vi "PolyCopyDocumentation.vi"   [LabVIEW 2020]
types:
  T1 = cluster{"VIPath":path, "Menu Name":string, "Selector Name":string}[]
  T2 = cluster{"vi reference":refnum<vi>, "Ctrls[]":refnum<vi>[]}
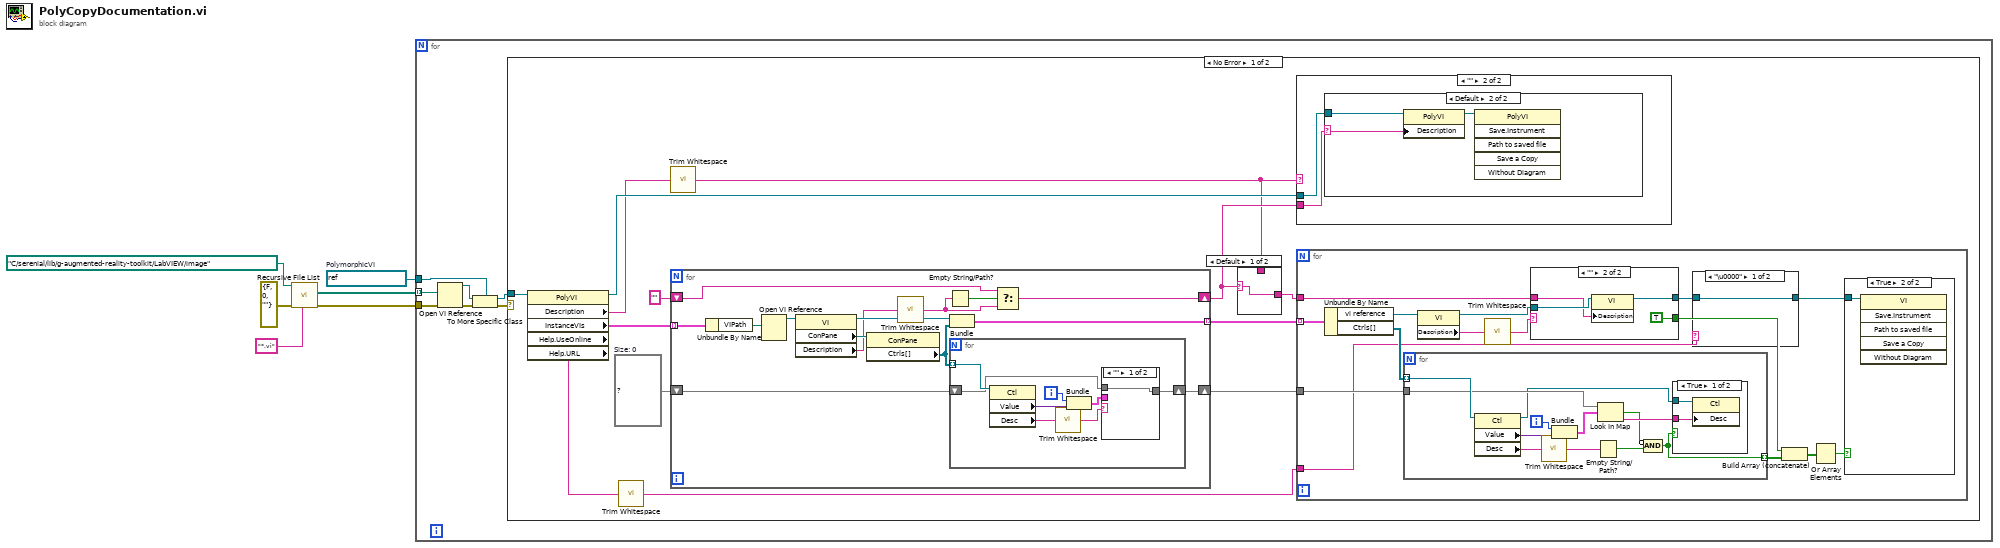
[diagram p0: block diagram]
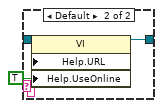
[diagram p5: hidden frame]
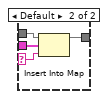
[diagram p9: hidden frame]
diagram:
  w3 = refnum<vi> refnum  # PolymorphicVI
  n1 = call <vilib>:"Recursive File List.vi"("pattern"="*.vi", "error in (no error)"=errorcluster {"status"=FALSE, "code"=0, "source"=""} ("error out"), "Folder Path"=path "C:/serenial/lib/g-augmented-reality-toolkit/LabVIEW/image") -> ("error out"=w6:errorcluster, "All Files in Dir"=w5:path[])  [unwired: 4 in, 3 out]
  n2 = for {
    tunnel: w6 -> [w13]
    tunnel: w5 -> [w12] mode=indexing
    tunnel: w3 -> [w11]
    n3 = Open VI Reference(vi path=w12, error in (no error)=w13) -> (vi reference=w10:refnum<vi>, error out=w9:errorcluster)  [unwired: 4 in]
    n4 = To More Specific Class(target class=w11, reference=w10, error in=w9) -> (specific class reference=w7:refnum<vi>, error out=w8:errorcluster)
    n5 = case shown="No Error" w8 {
      tunnel: w7 -> [w26 _]
      frame No Error {
        w25 = map{cluster{i32, "Value":variant}, string} {}  # Size: 0
        n6 = property class="PolyVI" props=["Description", "InstanceVIs", "Help.UseOnline", "Help.URL"](reference=w26) -> (reference out=w21:refnum<vi>, "Description"=w19:string, "InstanceVIs"=w20:T1, "Help.URL"=w15:string)  [unwired: 1 in, 2 out]
        n7 = call <vilib>:"Trim Whitespace.vi"("string"=w15) -> ("trimmed string"=w14:string)  [unwired: 1 in]
        n8 = call <vilib>:"Trim Whitespace.vi"("string"=w19) -> ("trimmed string"=w16:string)  [unwired: 1 in]
        n9 = for {
          tunnel: w20 -> [w87] mode=indexing
          shift-right: [w84] -> w22
          shift-left: w25 -> [w83]
          shift-right: [w75] -> w18
          shift-left: "" ("Description") -> [w77]
          tunnel: [w74] -> w23 mode=indexing
          n10 = Unbundle By Name(w87) -> ("VIPath"=w82:path)
          n11 = Open VI Reference(vi path=w82) -> (vi reference=w86:refnum<vi>)  [unwired: 5 in, 1 out]
          n12 = property class="VI"(reference=w86) -> (reference out=w81:refnum<vi>, "ConPane"=w85:refnum<vi>, "Description"=w79:string)  [unwired: 1 in, 1 out]
          n13 = property class="ConPane"(reference=w85) -> ("Ctrls[]"=w80:refnum<vi>[])  [unwired: 1 in, 2 out]
          n14 = call <vilib>:"Trim Whitespace.vi"("string"=w79) -> ("trimmed string"=w76:string)  [unwired: 1 in]
          n15 = Empty String/Path?(string/path=w76) -> (empty?=w78:bool)
          n16 = Bundle("vi reference"=w81, "Ctrls[]"=w80) -> (w74:T2)  [unwired: 1 in]
          n17 = for {
            tunnel: w80 -> [w95] mode=indexing
            shift-right: [w89] -> w84
            shift-left: w83 -> [w88]
            i -> [w93]
            n18 = property class="Ctl"(reference=w95) -> ("Value"=w94:variant, "Desc"=w91:string)  [unwired: 1 in, 2 out]
            n19 = call <vilib>:"Trim Whitespace.vi"("string"=w91) -> ("trimmed string"=w90:string)  [unwired: 1 in]
            n20 = Bundle(w93, "Value"=w94) -> (w92:cluster{i32, "Value":variant})  [unwired: 1 in]
            n21 = case shown="\"\"" w90 {
              selector: w90 -> [_ w99]
              tunnel: w92 -> [_ w100]
              tunnel: [w96 w98] -> w89
              tunnel: w88 -> [w96 w97]
              frame "" {
              }
              frame Default {
                n22 = Insert Into Map(map in=w97, key=w100, value=w99) -> (map out=w98:map{cluster{i32, "Value":variant}, string})  [unwired: 2 out]
              }
            }
          }
          n23 = Select(t=w77, s=w78, f=w76) -> (s? t:f=w75:string)
        }
        n24 = case shown="Default" w18 {
          selector: w18 -> [w27 _]
          tunnel: [w27 w28] -> w17
          tunnel: w16 -> [_ w28]
          frame Default {
          }
          frame "" {
          }
        }
        n25 = case shown="\"\"" w16 {
          tunnel: w21 -> [_ w30]
          tunnel: w18 -> [_ w29]
          frame Default {
          }
          frame "" {
            n26 = case shown="Default" w29 {
              selector: w29 -> [_ w32]
              tunnel: w30 -> [_ w33]
              frame "" {
              }
              frame Default {
                n27 = property class="PolyVI"(reference=w33, "Description"=w32) -> (reference out=w31:refnum<vi>)  [unwired: 1 in, 1 out]
                n28 = invoke class="PolyVI" method="Save.Instrument"(reference=w31) -> ()  [unwired: 5 in, 6 out]
              }
            }
          }
        }
        n29 = for {
          tunnel: w23 -> [w48] mode=indexing
          tunnel: w22 -> [w45]
          tunnel: w17 -> [w40]
          tunnel: w14 -> [w34]
          n30 = Unbundle By Name(w48) -> ("vi reference"=w47:refnum<vi>, "Ctrls[]"=w46:refnum<vi>[])
          n31 = for {
            tunnel: w46 -> [w71] mode=indexing
            tunnel: w45 -> [w68]
            tunnel: [w60] -> w38 mode=indexing
            i -> [w69]
            n32 = property class="Ctl"(reference=w71) -> (reference out=w65:refnum<vi>, "Value"=w70:variant, "Desc"=w64:string)  [unwired: 1 in, 1 out]
            n33 = call <vilib>:"Trim Whitespace.vi"("string"=w64) -> ("trimmed string"=w63:string)  [unwired: 1 in]
            n34 = Bundle(w69, "Value"=w70) -> (w67:cluster{i32, "Value":variant})  [unwired: 1 in]
            n35 = Empty String/Path?(string/path=w63) -> (empty?=w61:bool)
            n36 = Look In Map(map=w68, key=w67) -> (key not found?=w62:bool, value=w66:string)  [unwired: 1 in]
            n37 = Compound Arithmetic op=AND(invert w62, w61) -> (w60:bool)
            n38 = case shown="True" w60 {
              tunnel: w66 -> [w72 _]
              tunnel: w65 -> [w73 _]
              frame True {
                n39 = property class="Ctl"(reference=w73, "Desc"=w72) -> ()  [unwired: 1 in, 2 out]
              }
              frame False {
              }
            }
          }
          n40 = property class="VI"(reference=w47) -> (reference out=w41:refnum<vi>, "Description"=w44:string)  [unwired: 1 in, 1 out]
          n41 = call <vilib>:"Trim Whitespace.vi"("string"=w44) -> ("trimmed string"=w43:string)  [unwired: 1 in]
          n42 = case shown="\"\"" w43 {
            tunnel: [w55 w58] -> w42
            tunnel: w41 -> [w55 w59]
            tunnel: w40 -> [_ w57]
            tunnel: [_ TRUE] -> w39
            frame Default {
            }
            frame "" {
              n43 = property class="VI"(reference=w59, "Description"=w57) -> (reference out=w58:refnum<vi>)  [unwired: 1 in, 1 out]
            }
          }
          n44 = case shown="\"\"" w34 {
            selector: w34 -> [_ w51]
            tunnel: w42 -> [w49 w53]
            tunnel: [w49 w52] -> w35
            frame "\u0000" {
            }
            frame Default {
              n45 = property class="VI"(reference=w53, "Help.URL"=w51, "Help.UseOnline"=TRUE ("Help:Use Web URL")) -> (reference out=w52:refnum<vi>)  [unwired: 1 in, 1 out]
            }
          }
          n46 = Build Array (concatenate)(w39, w38) -> (w37:bool[])
          n47 = Or Array Elements(Boolean array=w37) -> (logical OR=w36:bool)
          n48 = case shown="True" w36 {
            tunnel: w35 -> [_ w54]
            frame False {
            }
            frame True {
              n49 = invoke class="VI" method="Save.Instrument"(reference=w54) -> ()  [unwired: 5 in, 6 out]
            }
          }
        }
      }
      frame Error {
      }
    }
  }
